vi "BuildZeroCue.vi"(1 "PXI card names":string[](array[string])=["DIO:", "6509", "Counter:", "6733_1", "Slow AO:", "6723", "Fast AO:", "6733_1", "6733_2", "6733_3"], 2 "Task cluster":T1={"inbits"=8, "outbits"=38, "Counter"="Counter", "Inbits"="Inbits", "Outbits"="Outbits", "Fast AO"=["FastAO_1", "FastAO_2", "FastAO_3"], "Errors"={"status"=FALSE, "code"=0, "source"=""}}) -> (0 "Zero Cue":T2[](array[typedef])=[{"Macro Instructions"=[], "Slow AO Array"=[{"ao line"="ao0", "Duration, Gain, NewVal"=[0.1, 1.0, 0.0, 0.0, 0.0]}, {"ao line"="ao1", "Duration, Gain, NewVal"=[0.1, 1.0, 0.0, 0.0, 0.0]}, {"ao line"="ao2", "Duration, Gain, NewVal"=[0.1, 1.0, 0.0, 0.0, 0.0]}, {"ao line"="ao3", "Duration, Gain, NewVal"=[0.1, 1.0, 0.0, 0.0, 0.0]}, {"ao line"="ao4", "Duration, Gain, NewVal"=[0.1, 1.0, 0.0, 0.0, 0.0]}, {"ao line"="ao5", "Duration, Gain, NewVal"=[0.1, 1.0, 0.0, 0.0, 0.0]}, {"ao line"="ao6", "Duration, Gain, NewVal"=[0.1, 1.0, 0.0, 0.0, 0.0]}, {"ao line"="ao7", "Duration, Gain, NewVal"=[0.1, 1.0, 0.0, 0.0, 0.0]}, {"ao line"="ao8", "Duration, Gain, NewVal"=[0.1, 1.0, 0.0, 0.0, 0.0]}, {"ao line"="ao9", "Duration, Gain, NewVal"=[0.1, 1.0, 0.0, 0.0, 0.0]}, {"ao line"="ao10", "Duration, Gain, NewVal"=[0.1, 1.0, 0.0, 0.0, 0.0]}, {"ao line"="ao11", "Duration, Gain, NewVal"=[0.1, 1.0, 0.0, 0.0, 0.0]}, {"ao line"="ao12", "Duration, Gain, NewVal"=[0.1, 1.0, 0.0, 0.0, 0.0]}, {"ao line"="ao13", "Duration, Gain, NewVal"=[0.1, 1.0, 0.0, 0.0, 0.0]}, {"ao line"="ao14", "Duration, Gain, NewVal"=[0.1, 1.0, 0.0, 0.0, 0.0]}, {"ao line"="ao15", "Duration, Gain, NewVal"=[0.1, 1.0, 0.0, 0.0, 0.0]}, {"ao line"="ao16", "Duration, Gain, NewVal"=[0.1, 1.0, 0.0, 0.0, 0.0]}, {"ao line"="ao17", "Duration, Gain, NewVal"=[0.1, 1.0, 0.0, 0.0, 0.0]}, {"ao line"="ao18", "Duration, Gain, NewVal"=[0.1, 1.0, 0.0, 0.0, 0.0]}, {"ao line"="ao19", "Duration, Gain, NewVal"=[0.1, 1.0, 0.0, 0.0, 0.0]}, {"ao line"="ao20", "Duration, Gain, NewVal"=[0.1, 1.0, 0.0, 0.0, 0.0]}, {"ao line"="ao21", "Duration, Gain, NewVal"=[0.1, 1.0, 0.0, 0.0, 0.0]}, {"ao line"="ao22", "Duration, Gain, NewVal"=[0.1, 1.0, 0.0, 0.0, 0.0]}, {"ao line"="ao23", "Duration, Gain, NewVal"=[0.1, 1.0, 0.0, 0.0, 0.0]}, {"ao line"="ao24", "Duration, Gain, NewVal"=[0.1, 1.0, 0.0, 0.0, 0.0]}, {"ao line"="ao25", "Duration, Gain, NewVal"=[0.1, 1.0, 0.0, 0.0, 0.0]}, {"ao line"="ao26", "Duration, Gain, NewVal"=[0.1, 1.0, 0.0, 0.0, 0.0]}, {"ao line"="ao27", "Duration, Gain, NewVal"=[0.1, 1.0, 0.0, 0.0, 0.0]}, {"ao line"="ao28", "Duration, Gain, NewVal"=[0.1, 1.0, 0.0, 0.0, 0.0]}, {"ao line"="ao29", "Duration, Gain, NewVal"=[0.1, 1.0, 0.0, 0.0, 0.0]}, {"ao line"="ao30", "Duration, Gain, NewVal"=[0.1, 1.0, 0.0, 0.0, 0.0]}, {"ao line"="ao31", "Duration, Gain, NewVal"=[0.1, 1.0, 0.0, 0.0, 0.0]}], "Duration (s)"=0.1, "Toggle"=TRUE}, {"Macro Instructions"=[{"Duration (s)"=0.1, "Steps"=1, "Changes"=[TRUE, TRUE, TRUE], "Triggers"=[FALSE, FALSE, FALSE, FALSE, FALSE, FALSE, FALSE, FALSE, FALSE, FALSE, FALSE, FALSE, FALSE, FALSE, FALSE, FALSE, FALSE, FALSE, FALSE, FALSE, FALSE, FALSE, FALSE, FALSE, FALSE, FALSE, FALSE, FALSE, FALSE, FALSE, FALSE, FALSE, FALSE, FALSE, FALSE, FALSE, FALSE, FALSE], "RAW cmds 2D"=[[0, 0, 0, 0, 0, 0, 0, 0], [0, 0, 0, 0, 0, 0, 0, 0], [0, 0, 0, 0, 0, 0, 0, 0]]}], "Slow AO Array"=[], "Duration (s)"=0.1, "Toggle"=FALSE}] {"Slow AO Array"."Duration, Gain, NewVal" format="%#_3g"})   [LabVIEW 2018]
uses:
  ActionCluster.ctl
  Instructions_RT.ctl
  ParameterSubCluster.ctl
  Tasks_RT.ctl
panel:
  # "Tasks and errors"
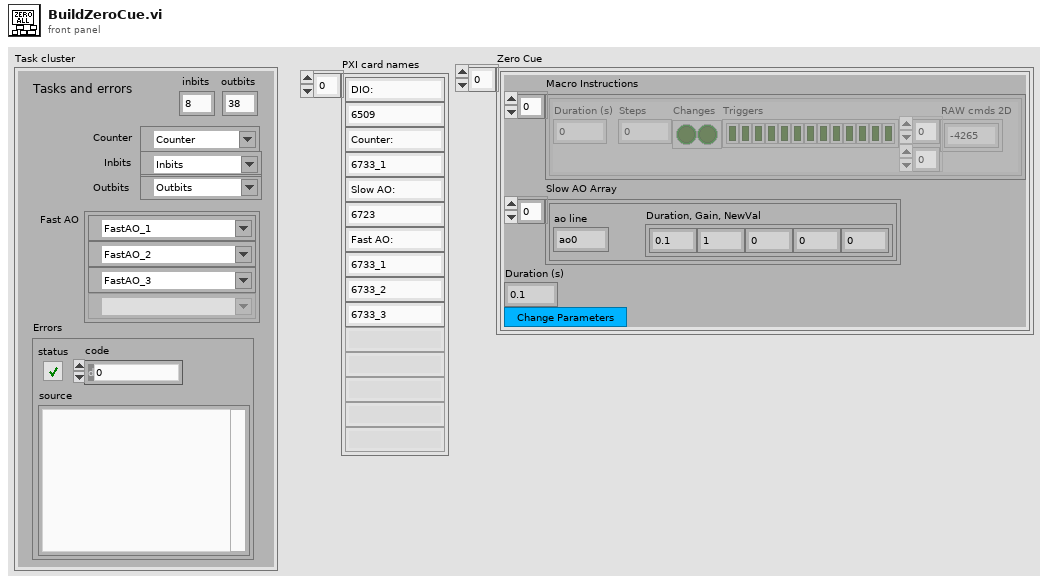
[diagram p1: front panel]
types:
  T1 = typedef "Tasks_RT.ctl" = cluster{"inbits":i32, "outbits":i32, "Counter":refnum<k21>, "Inbits":refnum<k21>, "Outbits":refnum<k21>, "Fast AO":refnum<k21>[], "Errors":errorcluster}
  T2 = typedef "ActionCluster.ctl" = cluster{"Macro Instructions":T3, "Slow AO Array":T4, "Duration (s)":dbl, "Toggle":bool}
  T3 = typedef "Instructions_RT.ctl" = cluster{"Duration (s)":dbl, "Steps":i32, "Changes":bool[], "Triggers":bool[], "RAW cmds 2D":i16[][]}[]
  T4 = typedef "ParameterSubCluster.ctl" = cluster{"ao line":string, "Duration, Gain, NewVal":dbl[]}[]
  T5 = cluster{"ao line":string, "Duration, Gain, NewVal":dbl[]}
  T6 = cluster{"Duration (s)":dbl, "Steps":i32, "Changes":bool[], "Triggers":bool[], "RAW cmds 2D":i16[][]}
  T7 = cluster{"Duration (s)":dbl, "Steps":i32, "Changes":bool[], "Triggers":bool[], "RAW cmds 2D":i16[][]}[]
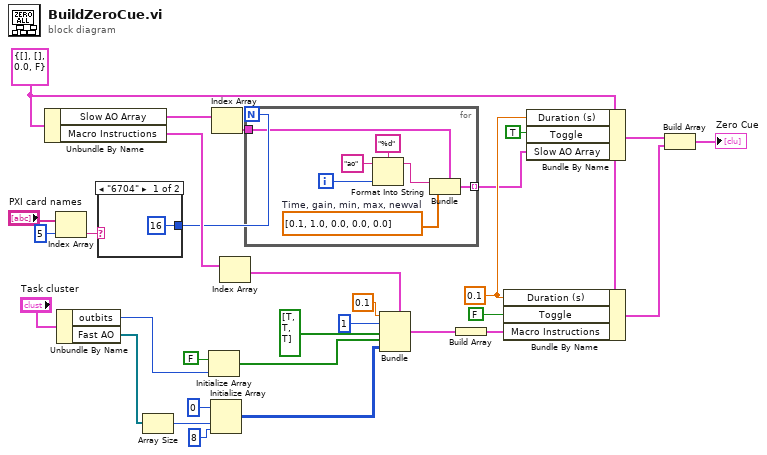
[diagram p0: block diagram]
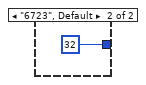
[diagram p2: hidden frame]
diagram:
  w28 = T2 {"Macro Instructions"=[], "Slow AO Array"=[], "Duration (s)"=0.0, "Toggle"=FALSE} ("element")
  w27 = 0.1 ("Duration (s)")
  n1 = Unbundle By Name(w28) -> ("Slow AO Array"=w23:T4, "Macro Instructions"=w22:T3)
  n2 = Index Array(array="PXI card names", index=5) -> (element=w6:string)
  n3 = Unbundle By Name("Task cluster") -> ("outbits"=w3:i32, "Fast AO"=w2:refnum<k21>[])
  n4 = case shown="\"6704\"" w6 {
    tunnel: [16 ("slow AO lines") 32 ("slow AO lines")] -> w5
    frame "6704" {
    }
    frame "6723", Default {
    }
  }
  n5 = Array Size(array=w2) -> (size(s)=w1:i32)
  n6 = Initialize Array(FALSE, w3) -> (w16:bool[])
  n7 = Initialize Array(i16 0 ("RAW cmds 2D"), w1, 8 ("dimension size")) -> (w13:i16[][])
  n8 = Index Array(array=w23) -> (element=w10:T5)  [unwired: 1 in]
  n9 = Index Array(array=w22) -> (element=w21:T6)  [unwired: 1 in]
  n10 = for {
    N: w5 -> [_]
    tunnel: w10 -> [w36]
    tunnel: [w33] -> w9 mode=indexing
    i -> [w39]
    w34 = dbl[] [0.1, 1.0, 0.0, 0.0, 0.0]  # Time, gain, min, max, newval
    n11 = Format Into String(format string="%d", initial string="ao", w39) -> (resulting string=w35:string)  [unwired: 1 in, 1 out]
    n12 = Bundle(cluster=w36, "ao line"=w35, "Duration, Gain, NewVal"=w34) -> (w33:T5)
  }
  n13 = Bundle(cluster=w21, "Duration (s)"=0.1, "Steps"=1, "Changes"=bool[] [TRUE, TRUE, TRUE], "Triggers"=w16, "RAW cmds 2D"=w13) -> (w12:T6)
  n14 = Build Array(w12) -> (w11:T7)
  n15 = Bundle By Name(cluster=w28, "Duration (s)"=w27, "Toggle"=FALSE, "Macro Instructions"=w11) -> (w29:T2)
  n16 = Bundle By Name(cluster=w28, "Duration (s)"=w27, "Toggle"=TRUE, "Slow AO Array"=w9) -> (w30:T2)
  n17 = Build Array(w30, w29) -> (→"Zero Cue":T2[])
